vi "ImageCalibration_subVi.vi"(8 "error in (no error)":errorcluster, 10 "Grid Descriptor":cluster{"X Step":sgl, "Y Step":sgl, "Unit":T1}, 11 "Preprocedded Img In":T4) -> (0 "error out":errorcluster, 1 "Error Map":sgl[][](array[numeric]) format="%.2f", 2 "Error Statistics":T5, 3 "Calibration Template Image (duplicate)":T4, 4 "Calibration Axis Info":T3={"Origin Pixel"={"X"=0.0, "Y"=0.0}, "Angle Relative to Horizontal (deg)"=0.0, "X Axis Pixel"={"X"=0.0, "Y"=0.0}, "Axis Reference"=1} {"X Axis Pixel"."Y" format="%.2f"; "X Axis Pixel"."X" format="%.2f"; "Axis Reference" items=["Direct", "Indirect"]; "Angle Relative to Horizontal (deg)" format="%.2f"; "Origin Pixel"."Y" format="%.2f"; "Origin Pixel"."X" format="%.2f"}, 5 "Reference Points":T2)   [LabVIEW 2020]
doc: "Vi che stima i parametri di calibrazione da un set up specifico (inserire descriz setup!!!).\nCostanti inteerne: Inserire descrizione"
uses:
  <vilib>/vision/Calibration.llb/Error Statistics.ctl
  <vilib>/vision/Image Controls.llb/IMAQ Image.ctl
  <vilib>/vision/Calibration.llb/Calibration Reference Points.ctl
  <vilib>/vision/Calibration.llb/Distortion Model.ctl
  <vilib>/vision/Calibration.llb/Distortion Model Types.ctl
  <vilib>/vision/NI_Vision_Development_Module.lvlib
panel:
  out "Calibration Template":T4(plugin-control)
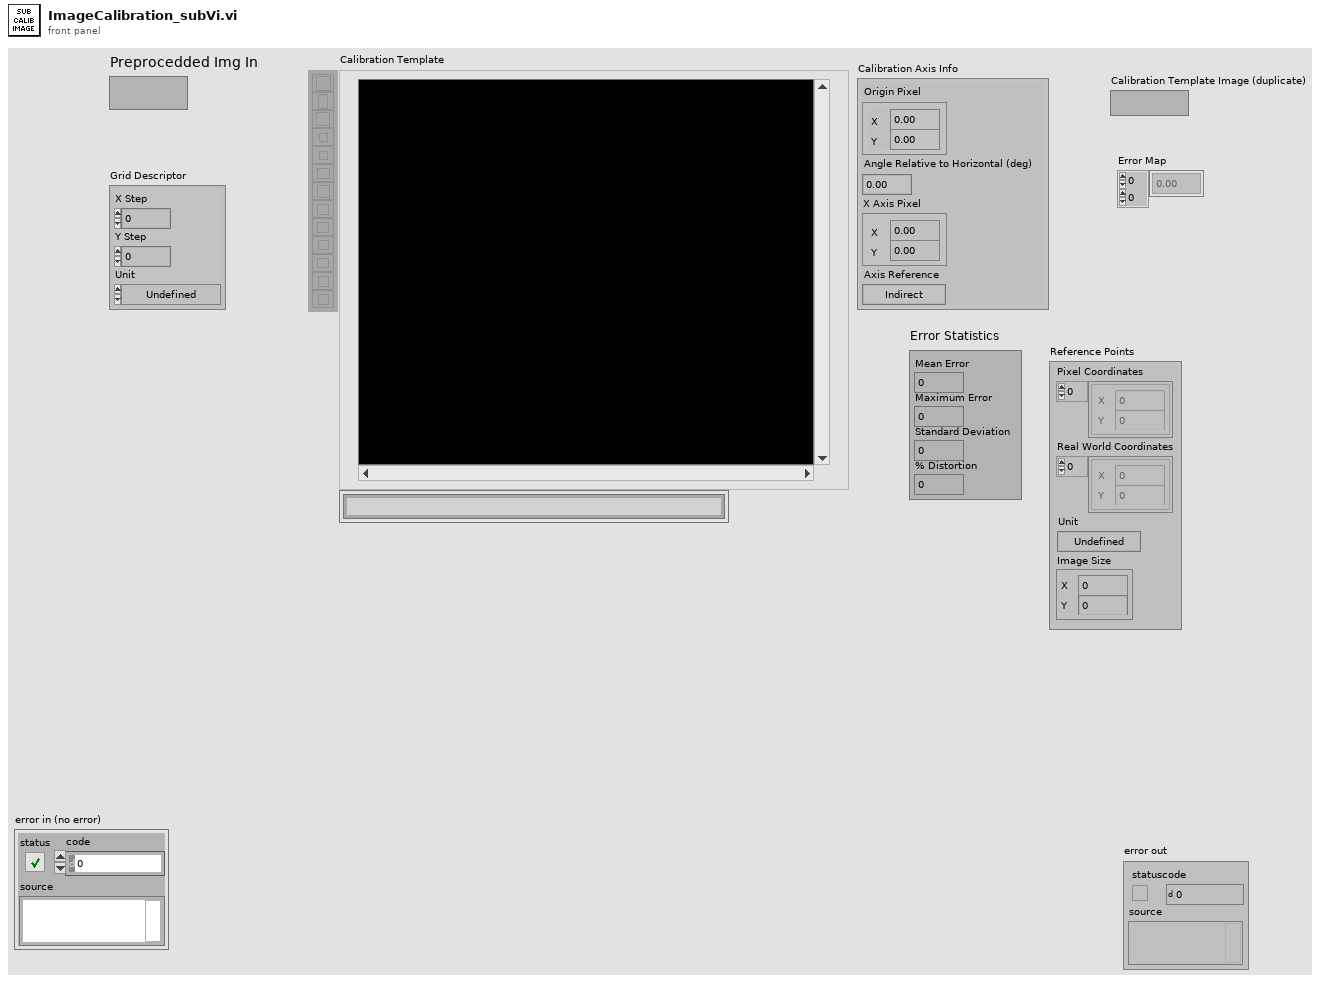
[diagram p1: front panel]
types:
  T1 = typedef "Image Unit" = enum32{"Undefined", "Angström", "Micrometer", "Millimeter", "Centimeter", "Meter", "Kilometer", "Microinch", "Inch", "Feet", "Nautical miles", "Standard miles", "Steps"}
  T2 = typedef "Calibration Reference Points.ctl" = cluster{"Pixel Coordinates":cluster{"X":dbl, "Y":dbl}[], "Real World Coordinates":cluster{"X":dbl, "Y":dbl}[], "Unit":T1, "Image Size":cluster{"X":u32, "Y":u32}}
  T3 = cluster{"Origin Pixel":cluster{"X":sgl, "Y":sgl}, "Angle Relative to Horizontal (deg)":sgl, "X Axis Pixel":cluster{"X":sgl, "Y":sgl}, "Axis Reference":u32}
  T4 = typedef "IMAQ Image.ctl" = refnum<image>
  T5 = typedef "Error Statistics.ctl" = cluster{"Mean Error":dbl, "Maximum Error":dbl, "Standard Deviation":dbl, "% Distortion":dbl}
  T6 = typedef "Distortion Model.ctl" = cluster{"Distortion Model":T7, "Polynomial Model Setup":cluster{"Radial Coefficient":u32, "Tangential Coefficients ":bool}}
  T7 = typedef "Distortion Model Types.ctl" = i32
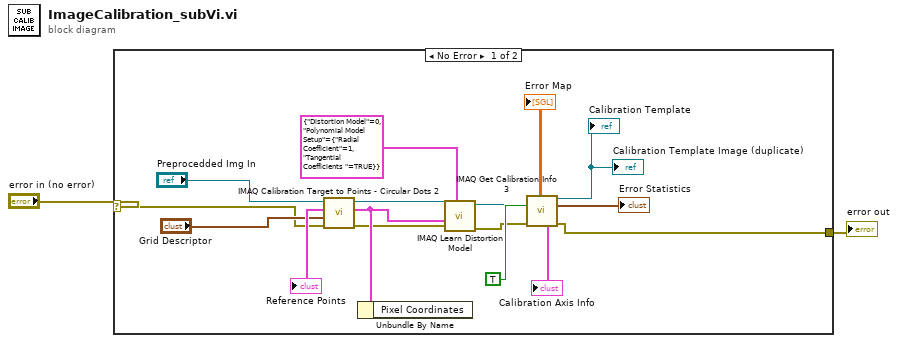
[diagram p0: block diagram]
diagram:
  n1 = case shown="No Error" "error in (no error)" {
    selector: "error in (no error)" -> [w4 w18]
    tunnel: [w3 w18] -> w1
    frame No Error {
      n2 = call "IMAQ Calibration Target to Points - Circular Dots 2"("error in (no error)"=w4, "Grid Descriptor"="Grid Descriptor", "Target Image"="Preprocedded Img In") -> ("error out"=w8:errorcluster, "Reference Points"=w9:T2, "Target Image (dup)"=w17:T4)  [unwired: 6 in]
      "Reference Points" <- w9
      n3 = Unbundle By Name(w9) -> ()  [unwired: 1 out]
      n4 = call "IMAQ Learn Distortion Model"("Distortion Model Setup"=T6 {"Distortion Model"=0, "Polynomial Model Setup"={"Radial Coefficient"=1, "Tangential Coefficients "=TRUE}}, "error in (no error)"=w8, "Reference Points"=w9, "Calibration Template Image"=w17) -> ("error out"=w12:errorcluster, "Calibration Template Image Out"=w13:T4)  [unwired: 6 in]
      n5 = call "IMAQ Get Calibration Info 3"("Calibration Template Image"=w13, "Return Error Information (False)"=TRUE, "error in (no error)"=w12) -> ("Error Map"=→"Error Map":sgl[][], "Calibration Template Image (duplicate)"=→"Calibration Template" →"Calibration Template Image (duplicate)":T4, "Error Statistics"=→"Error Statistics":T5, "Calibration Axis Info"=→"Calibration Axis Info":T3, "error out"=w3:errorcluster)  [unwired: 4 in, 4 out]
    }
    frame Error {
    }
  }
  "error out" <- w1
